vi "Hex Display.vi"(11 "Hex Display":string) -> (2 "Display":string, 3 "Normal Display":string)   [LabVIEW 2018]
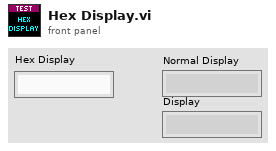
[diagram p1: front panel]
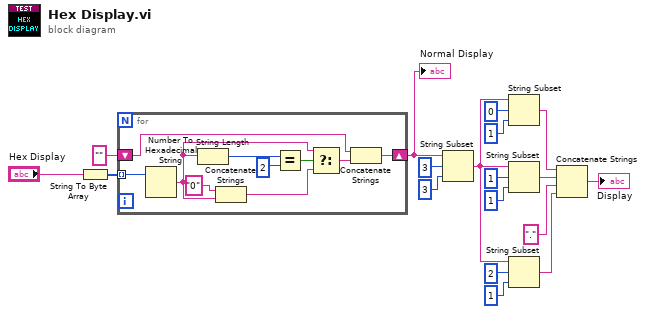
[diagram p0: block diagram]
diagram:
  n1 = String To Byte Array(string="Hex Display") -> (unsigned byte array=w17:u8[])
  n2 = for {
    tunnel: w17 -> [w28] mode=indexing
    shift-right: [w19] -> w15
    shift-left: "" -> [w20]
    n3 = Number To Hexadecimal String(2:w28) -> (0:w23:string)  [unwired: 1 in]
    n4 = String Length(string=w23) -> (length=w27:i32)
    n5 = Concatenate Strings("0" ("字符串"), w23) -> (w22:string)
    n6 = Equal?(x=w27, y=2) -> (x = y?=w24:bool)
    n7 = Select(t=w23, s=w24, f=w22) -> (s? t:f=w21:string)
    n8 = Concatenate Strings(w20, w21) -> (w19:string)
  }
  "Normal Display" <- w15
  n9 = String Subset(string=w15, offset (0)=3 ("偏移量(0)"), length (rest)=3 ("长度（剩余）")) -> (substring=w8:string)
  n10 = String Subset(string=w8, offset (0)=0 ("偏移量(0)"), length (rest)=1 ("长度（剩余）")) -> (substring=w5:string)
  n11 = String Subset(string=w8, offset (0)=1 ("偏移量(0)"), length (rest)=1 ("长度（剩余）")) -> (substring=w4:string)
  n12 = String Subset(string=w8, offset (0)=2 ("偏移量(0)"), length (rest)=1 ("长度（剩余）")) -> (substring=w1:string)
  n13 = Concatenate Strings(w5, w4, "." ("字符串"), w1) -> (→"Display":string)
